vi "New Data Point.vi"(8 "error in (no error)":errorcluster, 10 "X":dbl format="%#_13g", 11 "Linear in":refnum<class "Linear.lvclass">) -> (0 "error out":errorcluster, 2 "Y(X)":dbl, 3 "Linear out":refnum<class "Linear.lvclass">)   [LabVIEW 2020, in "Data Generators.lvlib" / "Linear.lvclass"]
uses:
  Linear.lvclass
  Linear.lvclass/Linear.ctl
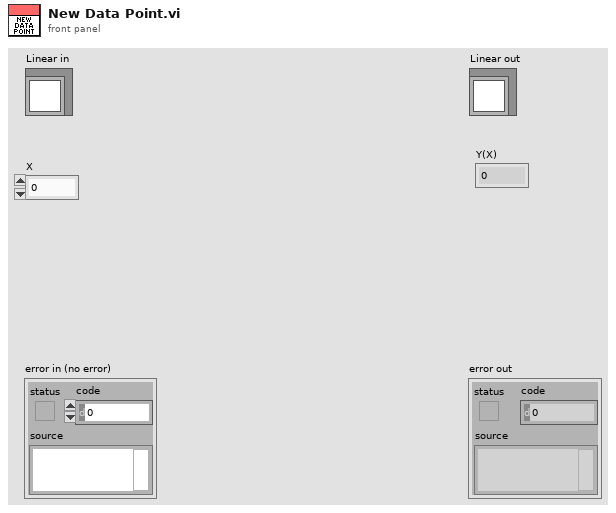
[diagram p1: front panel]
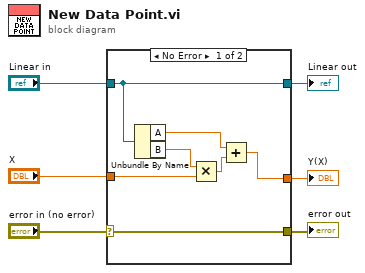
[diagram p0: block diagram]
diagram:
  n1 = case shown="No Error" "error in (no error)" {
    selector: "error in (no error)" -> [w13 w14]
    tunnel: [w13 w14] -> w5
    tunnel: "X" -> [w8 w16]
    tunnel: "Linear in" -> [w12 w15]
    tunnel: [w12 w15] -> w2
    tunnel: [w7 w16] -> w1
    frame No Error {
      n2 = Unbundle By Name(w12) -> ("A"=w11:dbl, "B"=w9:dbl)
      n3 = Multiply(x=w9, y=w8) -> (x*y=w10:dbl)
      n4 = Add(x=w11, y=w10) -> (x+y=w7:dbl)
    }
    frame Error {
    }
  }
  "error out" <- w5
  "Linear out" <- w2
  "Y(X)" <- w1
